vi "Rcv  Nested Content.vi"(8 "error in (no error)":errorcluster, 10 "Content":string, 11 "Root Actor in":refnum<class "Root Actor.lvclass">) -> (0 "error out":errorcluster, 3 "Root Actor out":refnum<class "Root Actor.lvclass">)   [LabVIEW 2020, in "Nested Actor.lvlib" / "Root Actor.lvclass"]
uses:
  Root Actor.lvclass
  Root Actor.lvclass/Root Actor.ctl
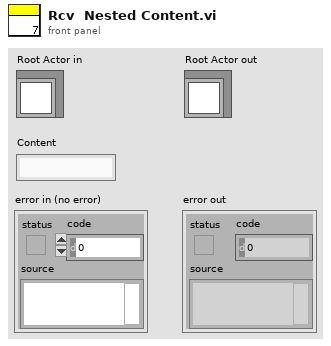
[diagram p1: front panel]
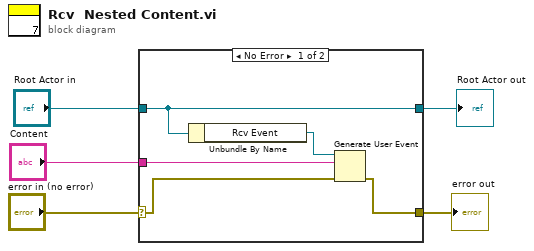
[diagram p0: block diagram]
diagram:
  n1 = case shown="No Error" "error in (no error)" {
    selector: "error in (no error)" -> [w7 w12]
    tunnel: [w6 w12] -> w4
    tunnel: [w10 w11] -> w2
    tunnel: "Root Actor in" -> [w10 w11]
    tunnel: "Content" -> [w8 _]
    frame No Error {
      n2 = Unbundle By Name(w10) -> ("Rcv Event"=w9:refnum<user-event>)
      n3 = Generate User Event(user event=w9, event data cluster=w8, error in=w7) -> (error out=w6:errorcluster)  [unwired: 1 in, 1 out]
    }
    frame Error {
    }
  }
  "error out" <- w4
  "Root Actor out" <- w2
